vi "Read VISA NXP.vi"(7 "Opciones":T1(ring), 8 "error in (no error)":errorcluster, 9 "Write":string, 10 "baud rate (9600)":u32=115200, 11 "VISA com port":refnum<visa-resource-name>) -> (0 "error out":errorcluster, 2 "Read":string, 3 "VISA com port 2":refnum<visa-resource-name>)   [LabVIEW 2020]
uses:
  <vilib>/Instr/_visa.llb/VISA Configure Serial Port (Instr).vi
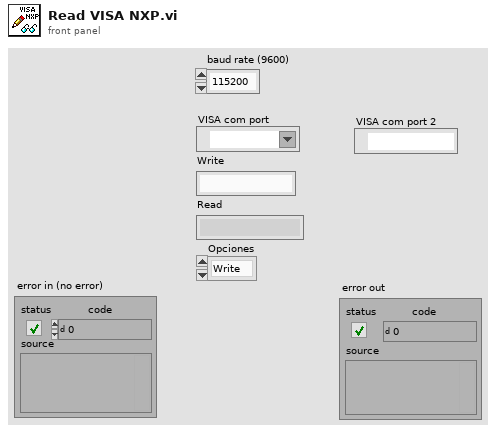
[diagram p1: front panel]
types:
  T1 = enum16{"Write", "Read", "Config", "Reset", "Close"}
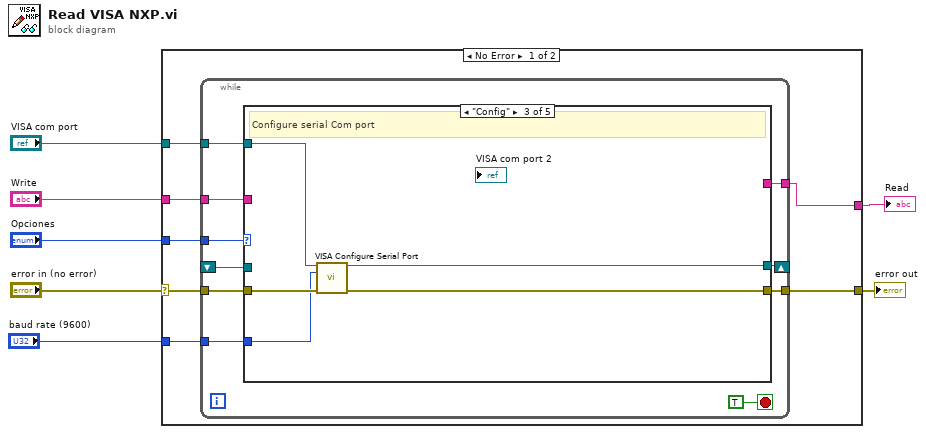
[diagram p0: block diagram]
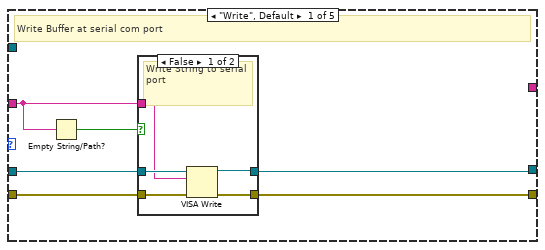
[diagram p2: hidden frame]
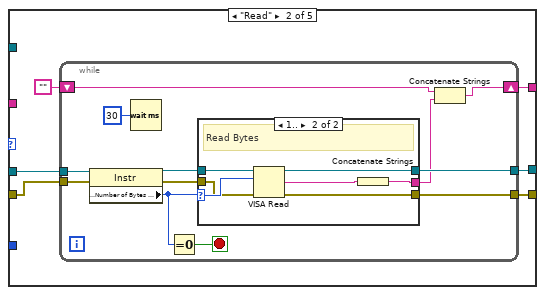
[diagram p4: hidden frame]
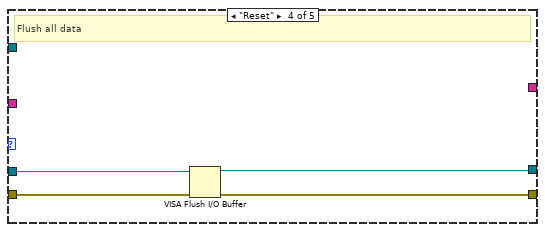
[diagram p6: hidden frame]
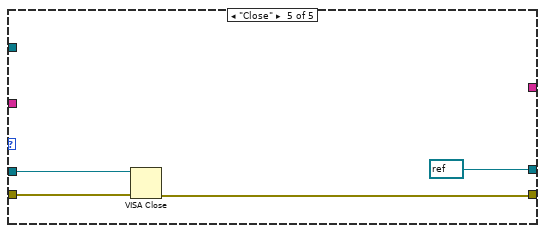
[diagram p7: hidden frame]
diagram:
  n1 = case shown="No Error" "error in (no error)" {
    selector: "error in (no error)" -> [w13 w78]
    tunnel: [w12 w78] -> w6
    tunnel: "Opciones" -> [w14 _]
    tunnel: "VISA com port" -> [w11 _]
    tunnel: "Write" -> [w10 _]
    tunnel: [w9 _] -> w2
    tunnel: "baud rate (9600)" -> [w8 _]
    frame No Error {
      n2 = while {
        tunnel: w14 -> [w23]
        tunnel: w13 -> [w22]
        tunnel: [w21] -> w12
        tunnel: w11 -> [w20]
        shift-right: [w19] -> _
        shift-left: _ -> [w18]
        tunnel: w10 -> [w17]
        tunnel: [w16] -> w9
        tunnel: w8 -> [w15]
        stop <- TRUE stop-if-true
        n3 = case shown="\"Config\"" w23 {
          tunnel: w22 -> [w30 w42 w69 w73 w77]
          tunnel: [w29 w41 w66 w72 w76] -> w21
          tunnel: w20 -> [_ _ w68 _ _]
          tunnel: [w25 w40 w67 w70 refnum<visa-resource-name> refnum ("VISA resource name out")] -> w19
          tunnel: w18 -> [w28 w43 _ w71 w75]
          tunnel: w17 -> [w27 _ _ _ _]
          tunnel: [_ w39 _ _ _] -> w16
          tunnel: w15 -> [_ _ w65 _ _]
          frame "Write", Default {
            # "Write Buffer at serial com port"
            n4 = Empty String/Path?(string/path=w27) -> (empty?=w26:bool)
            n5 = case shown="False" w26 {
              tunnel: w30 -> [w35 w36]
              tunnel: [w34 w36] -> w29
              tunnel: w28 -> [w33 w37]
              tunnel: w27 -> [w32 _]
              tunnel: [w31 w37] -> w25
              frame False {
                # "Write String to serial port"
                n6 = VISA Write(VISA resource name=w33, write buffer=w32, error in (no error)=w35) -> (VISA resource name out=w31:refnum<visa-resource-name>, error out=w34:errorcluster)  [unwired: 1 out]
              }
              frame True {
              }
            }
          }
          frame "Read" {
            n7 = while {
              tunnel: w43 -> [w55]
              tunnel: w42 -> [w54]
              tunnel: [w51] -> w41
              tunnel: [w50] -> w40
              shift-right: [w45] -> w39
              shift-left: "" -> [w44]
              stop <- w47 stop-if-true
              n8 = property class="Instr"(reference=w55, error in=w54) -> (reference out=w53:refnum<visa-resource-name>, error out=w52:errorcluster, "Serial Settings:Number of Bytes at Serial Port"=w48:u32)
              n9 = Wait (ms)(milliseconds to wait=u32 30) -> ()  [unwired: 1 out]
              n10 = Equal To 0?(x=w48) -> (x = 0?=w47:bool)
              n11 = case shown="1.." w48 {
                selector: w48 -> [_ w63]
                tunnel: w53 -> [w57 w64]
                tunnel: w52 -> [w56 w60]
                tunnel: [w56 w62] -> w51
                tunnel: [w57 w61] -> w50
                tunnel: [_ w58] -> w46
                frame 0, Default {
                }
                frame 1.. {
                  # "Read Bytes"
                  n12 = VISA Read(VISA resource name=w64, byte count=w63, error in (no error)=w60) -> (VISA resource name out=w61:refnum<visa-resource-name>, read buffer=w59:string, error out=w62:errorcluster)  [unwired: 1 out]
                  n13 = Concatenate Strings(w59) -> (w58:string)
                }
              }
              n14 = Concatenate Strings(w44, w46) -> (w45:string)
            }
          }
          frame "Config" {
            # "Configure serial Com port"
            n15 = call-poly "VISA Configure Serial Port"("VISA resource name"=w68, "baud rate (9600)"=w65, "error in (no error)"=w69) -> ("VISA resource name out"=w67:refnum<visa-resource-name>, "error out"=w66:errorcluster)  [unwired: 11 in]
          }
          frame "Reset" {
            # "Flush all data"
            n16 = VISA Flush I/O Buffer(VISA resource name=w71, error in (no error)=w73) -> (VISA resource name out=w70:refnum<visa-resource-name>, error out=w72:errorcluster)  [unwired: 1 in]
          }
          frame "Close" {
            n17 = VISA Close(VISA resource name=w75, error in (no error)=w77) -> (error out=w76:errorcluster)
          }
        }
      }
    }
    frame Error {
    }
  }
  "error out" <- w6
  "Read" <- w2
